vi "Day2ofPrison.vi"() -> ()   [LabVIEW 2017]
panel:
  in  "Stop Button":bool
  out "Waveform Graph 2":dynamicdata(graph)
  out "Waveform Graph":dynamicdata(graph)
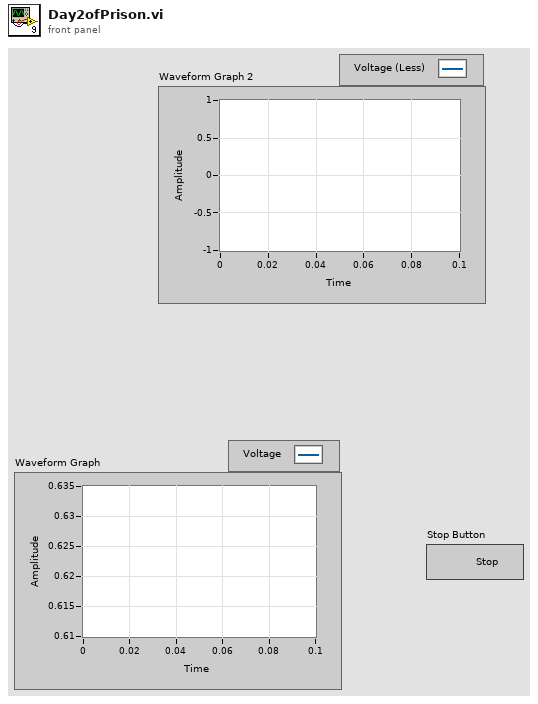
[diagram p1: front panel]
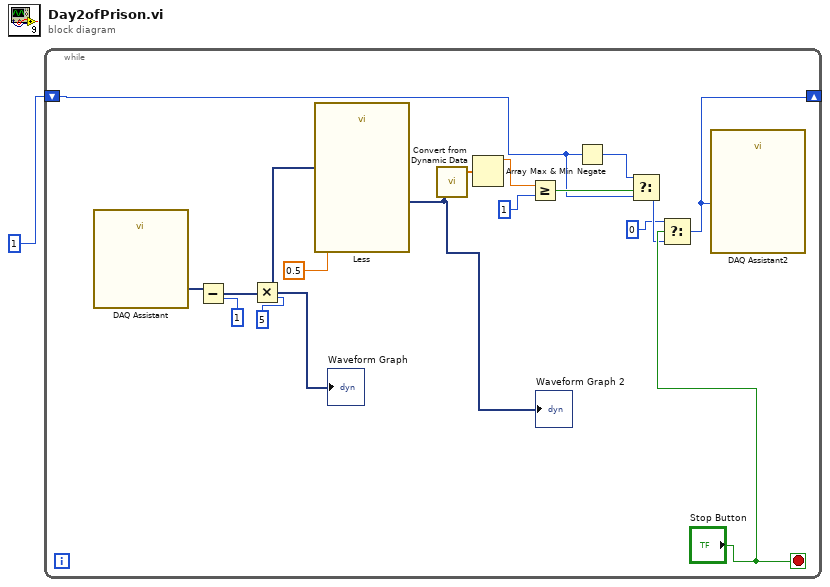
[diagram p0: block diagram]
diagram:
  n1 = while {
    shift-right: [w2] -> _
    shift-left: 1 -> [w6]
    stop <- "Stop Button" stop-if-true
    n2 = call "DAQ Assistant"() -> ("data"=w18:dynamicdata)  [unwired: 16 in, 3 out]
    n3 = Subtract(x=w18, y=1) -> (x-y=w17:dynamicdata)
    n4 = Multiply(x=w17, y=5) -> (x*y=w16:dynamicdata)
    "Waveform Graph" <- w16
    n5 = call "Less"("Constant Value to Compare Against"=0.5, "Operand 1"=w16) -> ("Result"=w12:dynamicdata)  [unwired: 8 in, 1 out]
    "Waveform Graph 2" <- w12
    n6 = call "Convert from Dynamic Data"("Dynamic Data Type"=w12) -> ("Array"=w11:dbl[])  [unwired: 3 in]
    n7 = Array Max & Min(array=w11) -> (max value=w10:dbl)  [unwired: 3 out]
    n8 = Greater Or Equal?(x=w10, y=1) -> (x >= y?=w8:bool)
    n9 = Negate(x=w6) -> (-x=w7:i32)
    n10 = Select(t=w7, s=w8, f=w6) -> (s? t:f=w4:i32)
    n11 = Select(t=0, s="Stop Button", f=w4) -> (s? t:f=w2:i32)
    n12 = call "DAQ Assistant2"("data"=w2) -> ()  [unwired: 17 in, 2 out]
  }
